vi "Collector.vi"() -> (1 "Lower Triggered?":bool, 2 "Upper Triggered?":bool)   [LabVIEW 2013]
doc: "Will Raise, Lower, or Stop the collector motor if a button is pressed for either, and will stop if hit by a limit switch."
uses:
  CollectorEnum.ctl
panel:
  in  "CollectorAction":T1
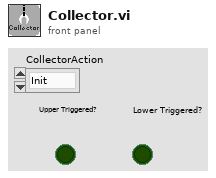
[diagram p1: front panel]
types:
  T1 = typedef "CollectorEnum.ctl" = enum16{"Init", "Raise", "Lower", "Stop", "GetStatus"}
  T2 = typedef "WPI_MotorControlDeviceRef.ctl" = cluster{"DeviceStatus":errorcluster, "Type":enum16{"PWM", "CAN"}, "PWM":cluster{"Digital Module":T3, "PWM Channel":T4, "DeadBand":T5}, "CAN":cluster{"Device Number":u8, "Control Mode":T6, "Semaphore":T7, "Max Vout":dbl}, "Invert":bool, "TransformRef":T8, "InvTransformRef":T8}
  T3 = typedef "FPGA_TypedefDigitalModule.ctl" = enum16{"Digital Module 1", "Digital Module 2"}
  T4 = typedef "FPGA_DIOPWMChannel.ctl" = enum8{"PWM 1", "PWM 2", "PWM 3", "PWM 4", "PWM 5", "PWM 6", "PWM 7", "PWM 8", "PWM 9", "PWM 10", "Invalid"}
  T5 = typedef "WPI_PWMDeadband.ctl" = cluster{"Name":string, "maxPositivePwm":i32, "minPositivePwm":i32, "centerPwm":i32, "maxNegativePwm":i32, "minNegativePwm":i32, "angularRange":u16}
  T6 = typedef "WPI_CANJaguar_ControlMode.ctl" = enum8{"Percent VBus", "Current", "Speed", "Position", "Voltage"}
  T7 = typedef "Semaphore RefNum" = refnum<k1>
  T8 = typedef "WPI_PWMTransform_ConPane.ctl" = refnum<vi>
  T9 = typedef "WPI_DigitalInputDevRef.ctl" = cluster{"DevStatus":errorcluster, "DIO Channel":T10, "Digital Module":T3}
  T10 = typedef "FPGA_DIOChannel.ctl" = enum8{"DIO 1", "DIO 2", "DIO 3", "DIO 4", "DIO 5", "DIO 6", "DIO 7", "DIO 8", "DIO 9", "DIO 10", "DIO 11", "DIO 12", "DIO 13", "DIO 14", "Invalid"}
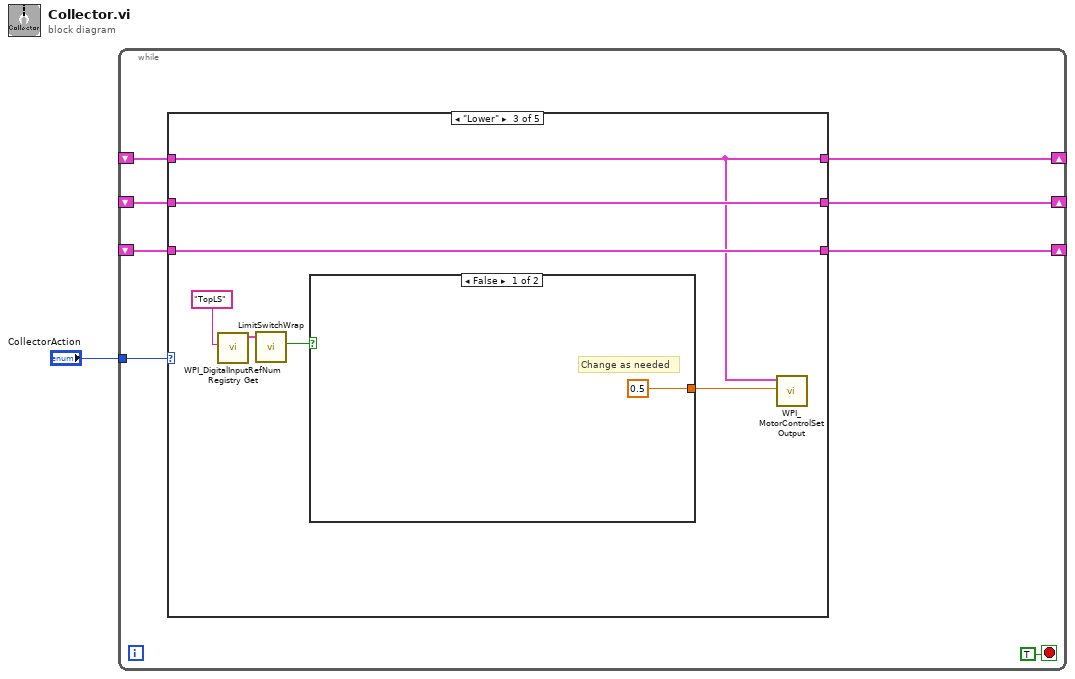
[diagram p0: block diagram]
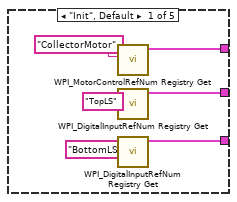
[diagram p2: hidden frame]
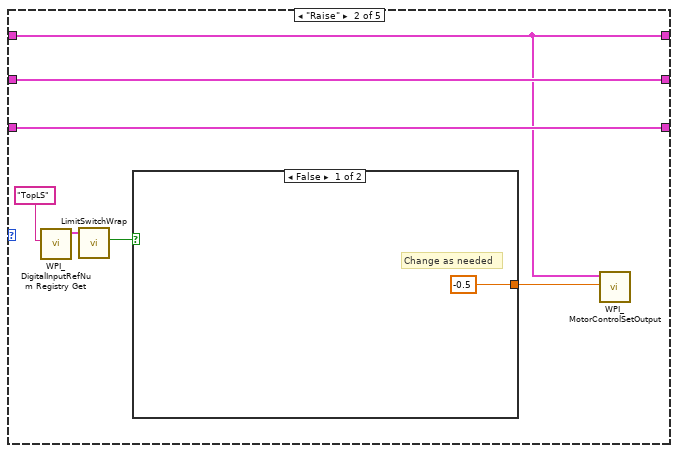
[diagram p3: hidden frame]
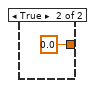
[diagram p4: hidden frame]
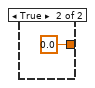
[diagram p5: hidden frame]
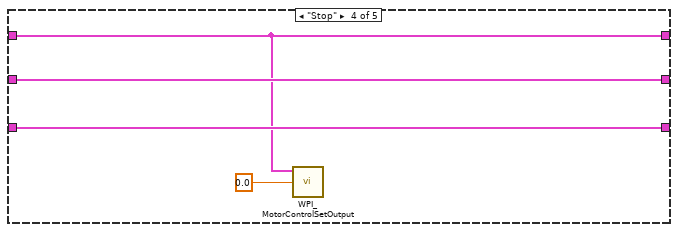
[diagram p6: hidden frame]
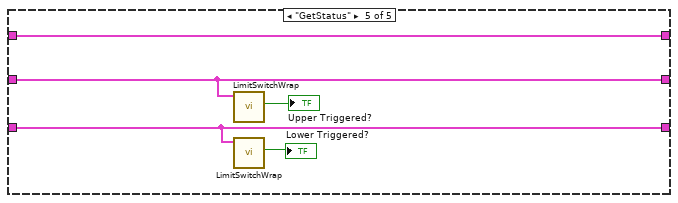
[diagram p7: hidden frame]
diagram:
  n1 = while {
    tunnel: "CollectorAction" -> [w9]
    shift-right: [w5] -> _
    shift-left: _ -> [w2]
    shift-right: [w6] -> _
    shift-left: _ -> [w3]
    shift-right: [w7] -> _
    shift-left: _ -> [w4]
    stop <- TRUE stop-if-true
    n2 = case shown="\"Lower\"" w9 {
      tunnel: [w12 w16 w25 w34 w42] -> w7
      tunnel: [w11 w18 w27 w36 w41] -> w6
      tunnel: [w10 w17 w26 w35 w40] -> w5
      tunnel: w4 -> [_ w16 w25 w34 w42]
      tunnel: w3 -> [_ w18 w27 w36 w41]
      tunnel: w2 -> [_ w17 w26 w35 w40]
      frame "Init", Default {
        n3 = call <vilib>:"WPI_MotorControlRefNum Registry Get.vi"("refnum name"="CollectorMotor") -> ("MotorControlDevRef"=w12:T2)  [unwired: 9 in, 1 out]
        n4 = call <vilib>:"WPI_DigitalInputRefNum Registry Get.vi"("refnum name"="TopLS") -> ("DigitalInputDevRef"=w11:T9)  [unwired: 9 in, 1 out]
        n5 = call <vilib>:"WPI_DigitalInputRefNum Registry Get.vi"("refnum name"="BottomLS") -> ("DigitalInputDevRef"=w10:T9)  [unwired: 9 in, 1 out]
      }
      frame "Raise" {
        n6 = call <vilib>:"WPI_DigitalInputRefNum Registry Get.vi"("refnum name"="TopLS") -> ("DigitalInputDevRef"=w20:T9)  [unwired: 9 in, 1 out]
        n7 = call "LimitSwitchWrap.vi"("DigitalInputDevRef"=w20) -> ("Triggered"=w22:bool)  [unwired: 9 in, 1 out]
        n8 = case shown="False" w22 {
          tunnel: [-0.5 0.0] -> w21
          frame False {
            # "Change as needed"
          }
          frame True {
          }
        }
        n9 = call <vilib>:"WPI_MotorControlSetOutput.vi"("Output"=w21, "MotorControlDevRef"=w16) -> ()  [unwired: 7 in, 3 out]
      }
      frame "Lower" {
        n10 = call <vilib>:"WPI_DigitalInputRefNum Registry Get.vi"("refnum name"="TopLS") -> ("DigitalInputDevRef"=w29:T9)  [unwired: 9 in, 1 out]
        n11 = call "LimitSwitchWrap.vi"("DigitalInputDevRef"=w29) -> ("Triggered"=w31:bool)  [unwired: 9 in, 1 out]
        n12 = case shown="False" w31 {
          tunnel: [0.5 0.0] -> w30
          frame False {
            # "Change as needed"
          }
          frame True {
          }
        }
        n13 = call <vilib>:"WPI_MotorControlSetOutput.vi"("Output"=w30, "MotorControlDevRef"=w25) -> ()  [unwired: 7 in, 3 out]
      }
      frame "Stop" {
        n14 = call <vilib>:"WPI_MotorControlSetOutput.vi"("Output"=0.0, "MotorControlDevRef"=w34) -> ()  [unwired: 7 in, 3 out]
      }
      frame "GetStatus" {
        n15 = call "LimitSwitchWrap.vi"("DigitalInputDevRef"=w41) -> ("Triggered"=→"Upper Triggered?":bool)  [unwired: 9 in, 1 out]
        n16 = call "LimitSwitchWrap.vi"("DigitalInputDevRef"=w40) -> ("Triggered"=→"Lower Triggered?":bool)  [unwired: 9 in, 1 out]
      }
    }
  }
